vi "Z900_navX_Internal_ProcessingLoop.vi"(11 "navX Device":T1={"Interface"={"Protocol"=enum."SERIAL", "Update Rate (4Hz-60Hz)"=4, "navX Open TypeDef"=variant}, "Notify Packet"=refnum, "Loop VI Refnum"=refnum, "Ready to Close Occurrence Refnum"=refnum} {"Interface"."Update Rate (4Hz-60Hz)" min=4 max=60 step=1}) -> (0 "error out":errorcluster, 2 "Registry":u8[](array[numeric]))   [LabVIEW 2017, in "navX Library v2.lvlib"]
doc: "This navX VI handles the reading/writing for the navX. All of the good stuff is in here.\nTHIS VI SHOULD NOT BE CALLED BY THE USER!"
uses:
  navX Library v2.lvlib
  TypeDefs/Z900_navX_DeviceTypeDef.ctl
  TypeDefs/Z900_navX_ProtocolTypeDef.ctl
  TypeDefs/Z900_navX_NotifyPacketTypeDef.ctl
  TypeDefs/Z900_navX_ActionTypeDef.ctl
  <vilib>/Platform/TimedLoop/XDataNode/timing_clust.ctl
  <vilib>/Platform/TimedLoop/XDataNode/nitl_modes.ctl
  <vilib>/Platform/TimedLoop/XDataNode/wakeup.ctl
  TypeDefs/navX Open TypeDefs/Z900_navX_OpenTypeDef_Serial.ctl
  NI WPI/WPI_SerialPort_USB.ctl
  TypeDefs/Z900_navX_SerialStreamTypeDef.ctl
  TypeDefs/Z900_navX_ZeroVectorTypeDef.ctl
  TypeDefs/Z900_navX_DeviceRegisters.ctl
  TypeDefs/Flags/Z900_navX_Flags_CapabilityTypeDef.ctl
  <vilib>/Rock Robotics/SystemInterfaces/Utilities/FPGA_UtilitiesRead LocalTime.vi
  <vilib>/Platform/TimedLoop/XDataNode/XDataNode.xnode
  <vilib>/Platform/TimedLoop/XDataNode/XDNodeRunTimeDep.lvlib
  NI WPI/NI WPI Serial USB.lvlib
panel:
  out "Connected":bool
  in  "Halt":bool
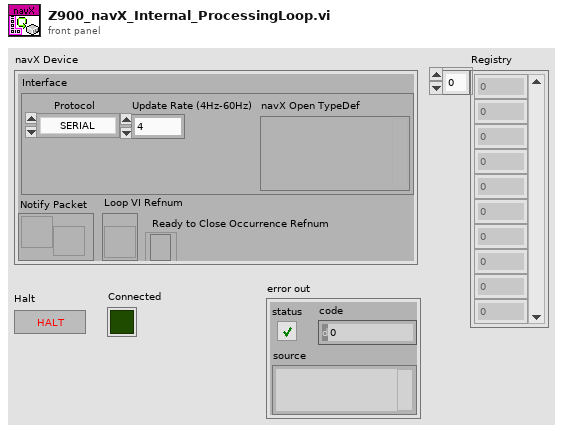
[diagram p1: front panel]
types:
  T1 = typedef "navX Library v2.lvlib/Z900_navX_DeviceTypeDef.ctl" = cluster{"Interface":cluster{"Protocol":T2, "Update Rate (4Hz-60Hz)":u8, "navX Open TypeDef":variant}, "Notify Packet":refnum<notifier>, "Loop VI Refnum":refnum<vi>, "Ready to Close Occurrence Refnum":refnum<k4>}
  T2 = typedef "navX Library v2.lvlib/Z900_navX_ProtocolTypeDef.ctl" = enum16{"SERIAL", "I2C", "SPI"}
  T3 = typedef "navX Library v2.lvlib/Z900_navX_InterfaceTypeDef.ctl" = cluster{"SerialPortRef":T4, "I2CDevRef":T5, "SPIDevRef":T7}
  T4 = typedef "WPI_SerialPortRef.ctl" = cluster{"DevStatus":errorcluster, "Serial Port Name":refnum<visa-resource-name>}
  T5 = typedef "WPI_I2CDevRef.ctl" = cluster{"DevStatus":errorcluster, "Device Address":u8, "Handle":i32, "I2C Bus":T6}
  T6 = typedef "i2c_bus.ctl" = enum16{"I2C On-Board", "I2C MXP", "Invalid"}
  T7 = typedef "WPI_SPIDevRef.ctl" = cluster{"DevStatus":errorcluster, "Handle":i32, "SPI Bus":T8}
  T8 = typedef "spi_bus.ctl" = enum16{"SPI On-Board, CS0", "SPI On-Board, CS1", "SPI On-Board, CS2", "SPI On-Board, CS3", "SPI MXP", "Invalid"}
  T9 = cluster{"Last Valid FPGA Time":dbl, "Error Count":i32, "Initialized":bool}
  T10 = typedef "XDNodeRunTimeDep.lvlib/timing_clust.ctl" = cluster{"Expected End [f-1]":u64, "Actual End [f-1]":u64, "Finished Late? [f-1]":bool, "Expected End [i-1]":u64, "Actual End [i-1]":u64, "Finished Late? [i-1]":bool, "Expected Start [i]":u64, "Actual Start [i]":u64, "Expected Start [f]":u64, "Actual Start [f]":u64, "Source Name":string, "Structure Name":string, "Period":i64, "Deadline":i64, "Offset":i64, "Start":i64, "Priority":i32, "Timeout":i32, "Mode":T11, "Wakeup Reason":T12, "Error":errorcluster, "Source Type":string, "Secondary Source Type":string, "Global End Time":u64, "Global Start Time":u64, "Frame Duration":u64, "Iteration Duration":u64, "Assigned CPU":i32, "I/O Scan Engine Mode":u32}
  T11 = typedef "XDNodeRunTimeDep.lvlib/nitl_modes.ctl" = enum32{"No Change", "Process missed periods, maintain original phase", "Discard missed periods, maintain original phase", "Process missed periods, ignore original phase", "Discard missed periods, ignore original phase"}
  T12 = typedef "XDNodeRunTimeDep.lvlib/wakeup.ctl" = enum32{"Normal", "Aborted", "Asynchronous wakeup", "Timing source error", "Timed loop error", "Timeout"}
  T13 = typedef "navX Library v2.lvlib/Z900_navX_OpenTypeDef_Serial.ctl" = cluster{"Serial Port":T14, "Stream Type":T15}
  T14 = typedef "NI WPI Serial USB.lvlib/WPI_SerialPort_USB.ctl" = enum16{"Onboard RS-232", "MXP TTL", "USB"}
  T15 = typedef "navX Library v2.lvlib/Z900_navX_SerialStreamTypeDef.ctl" = enum16{"YRPH", "Quaterinons", "Gyro/Raw", "AHRS", "AHRSAndPositioning"}
  T16 = typedef "navX Library v2.lvlib/Z900_navX_ZeroVectorTypeDef.ctl" = cluster{"X":bool, "Y":bool, "Z":bool}
  T17 = typedef "navX Library v2.lvlib/Z900_navX_NotifyPacketTypeDef.ctl" = cluster{"navX Action":T18, "Data":variant}
  T18 = typedef "navX Library v2.lvlib/Z900_navX_ActionTypeDef.ctl" = enum16{"None", "Halt", "Update Serial Protocol", "Zero-Yaw", "Zero-Displacement", "Zero-Velocity"}
  T19 = typedef "navX Library v2.lvlib/Z900_navX_DeviceRegisters.ctl" = u8
  T20 = typedef "navX Library v2.lvlib/Z900_navX_Flags_CapabilityTypeDef.ctl" = u16
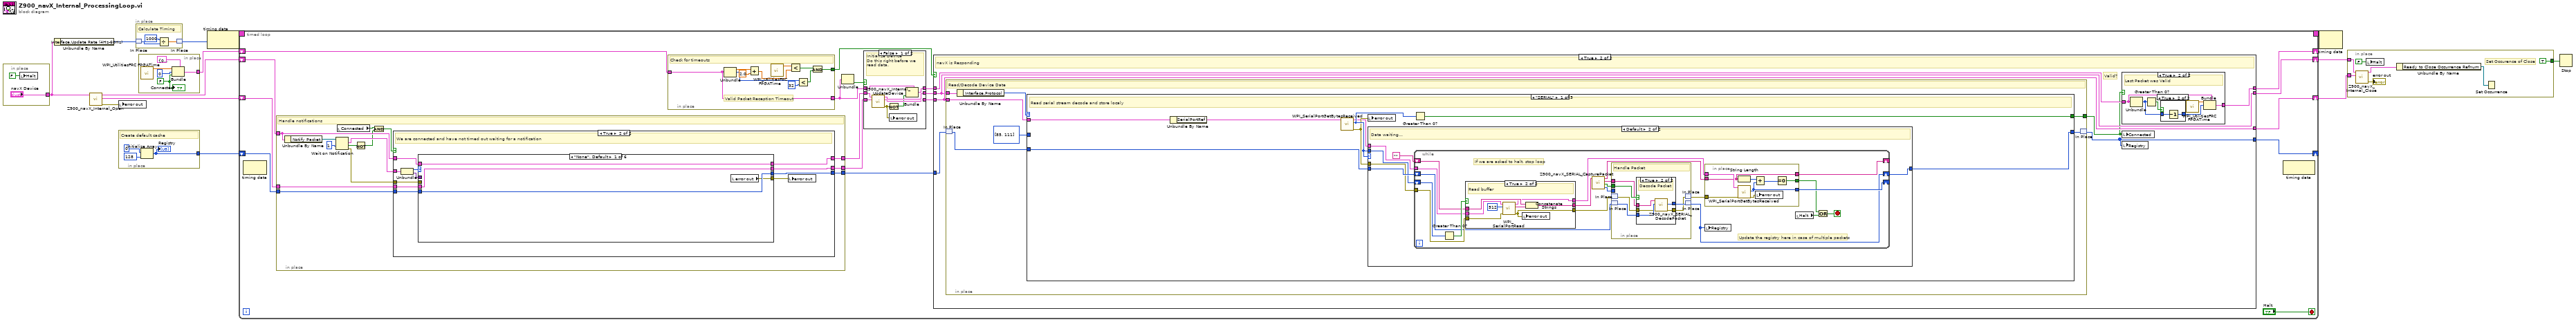
[diagram p0: block diagram]
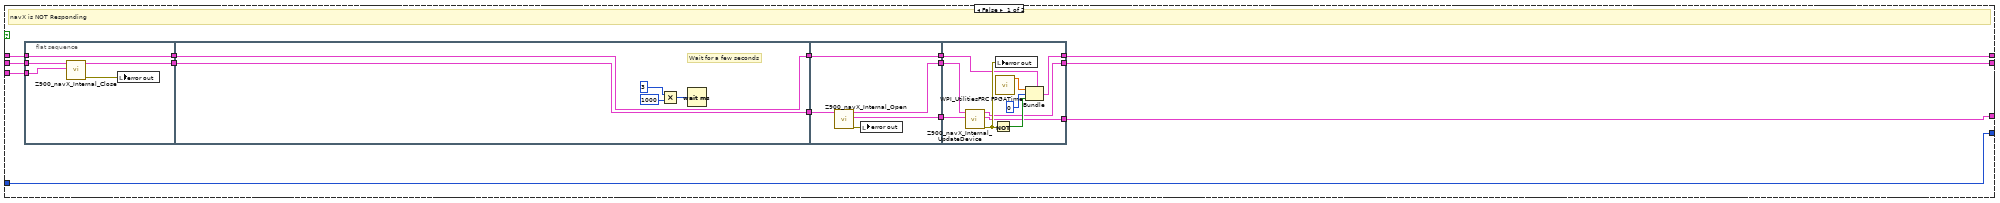
[diagram p3: hidden frame]
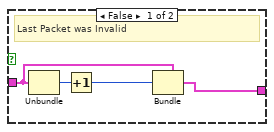
[diagram p4: hidden frame]
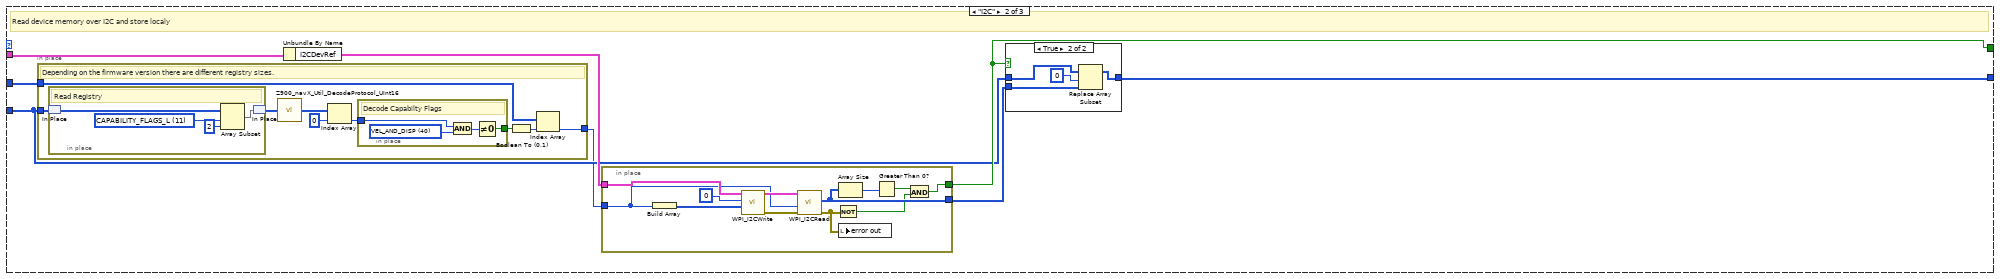
[diagram p9: hidden frame]
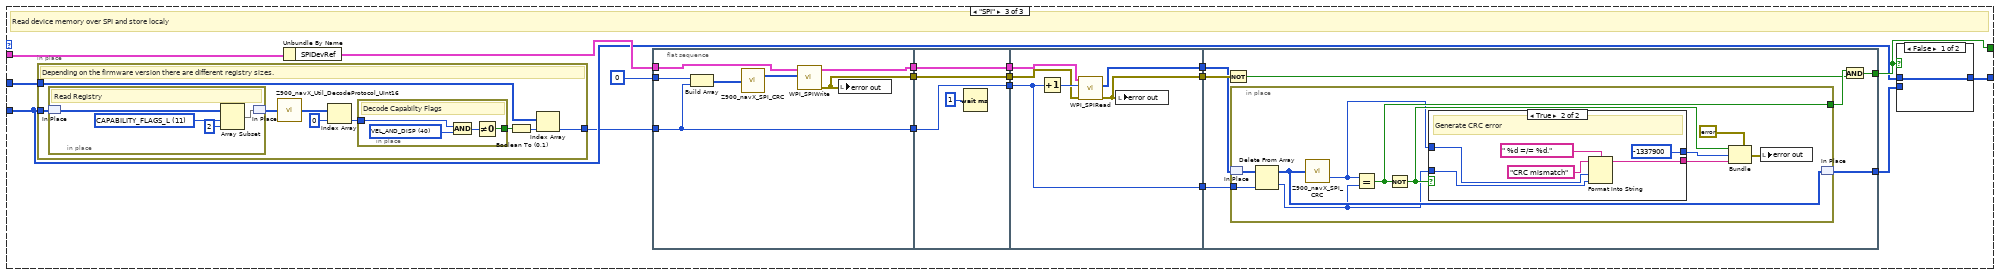
[diagram p11: hidden frame]
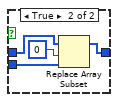
[diagram p12: hidden frame]
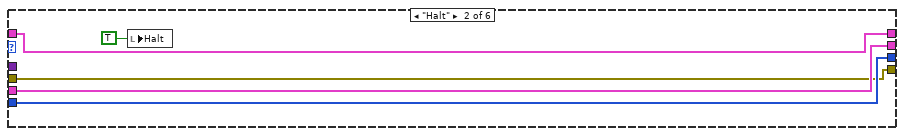
[diagram p15: hidden frame]
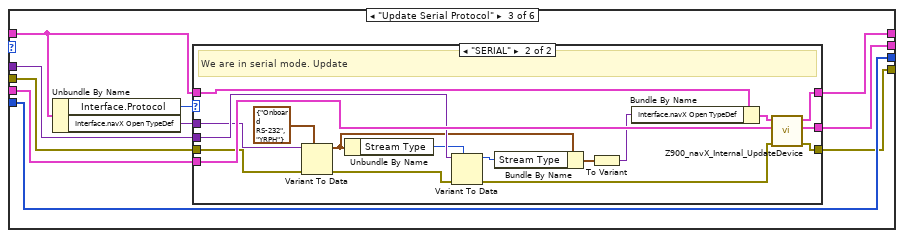
[diagram p16: hidden frame]
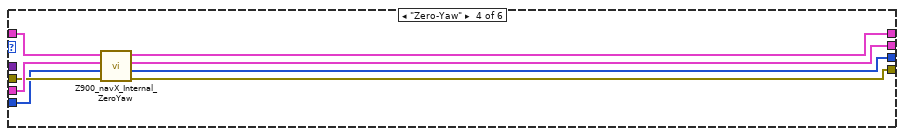
[diagram p18: hidden frame]
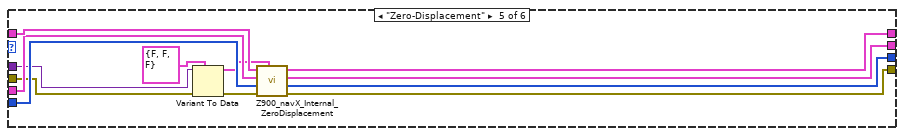
[diagram p19: hidden frame]
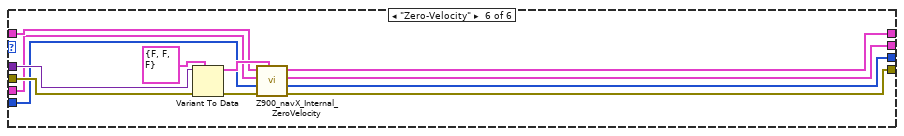
[diagram p20: hidden frame]
diagram:
  n1 = in-place {
    in-place-border: ["navX Device"] -> w6
    n2 = local write "Halt"(FALSE ("Halt")) -> ()
  }
  n3 = Unbundle By Name(w6) -> ("Interface.Update Rate (4Hz-60Hz)"=w10:u8)
  n4 = call "Z900_navX_Internal_Open.vi"("navX Device"=w6) -> ("error out"=w2:errorcluster, "Interface TypeDefs"=w5:T3, "navX Device"=w3:T1)  [unwired: 8 in]
  n5 = local write "error out"(w2) -> ()
  n6 = in-place {
    in-place-border: [w16] -> w9
    # "Create default cache"
    n7 = Initialize Array(u8 0 ("Received Data"), 128 ("hex")) -> (w16:u8[])
    "Registry" <- w16
  }
  n8 = in-place {
    # "Calculate Timing"
    n9 = in-place-match #1(w10) -> (w20:u8)
    n10 = Divide(x=1000, y=w20) -> (x/y=w19:dbl)
    n11 = in-place-match #1(w19) -> (w11:u8)
  }
  n12 = in-place {
    in-place-border: [w24] -> w4
    w22 = FALSE ("Initialized")
    n13 = call <vilib>:"WPI_UtilitiesFRC FPGATime.vi"() -> ("FPGA Time"=w25:dbl)  [unwired: 10 in, 1 out]
    n14 = Bundle(cluster=T9 {"Last Valid FPGA Time"=0.0, "Error Count"=0, "Initialized"=FALSE}, "Last Valid FPGA Time"=w25, "Error Count"=0, "Initialized"=w22) -> (w24:T9)
    "Connected" <- w22
  }
  n15 = node-c288(w11) -> (w13:T10)
  n16 = timed-loop {
    timing: w13 -> [_]
    timing-out: [_] -> w12
    shift-right: [w44] -> _
    shift-left: w9 -> [w40]
    shift-right: [w41] -> w8
    shift-left: w3 -> [w30]
    shift-right: [w42] -> w7
    shift-left: w5 -> [w29]
    shift-right: [w43] -> _
    shift-left: w4 -> [w27]
    stop <- "Halt" stop-if-true
    n17 = node-c288() -> ()  [unwired: 1 in, 1 out]
    n18 = in-place {
      in-place-border: w30 -> [w332]
      in-place-border: w29 -> [w331]
      in-place-border: [w330] -> w33
      in-place-border: [w329] -> w34
      in-place-border: w40 -> [w327]
      in-place-border: [w326] -> w39
      # "Handle notifications"
      n19 = Unbundle By Name(w332) -> ("Notify Packet"=w334:refnum<notifier>)
      n20 = Wait on Notification(notifier=w334, timeout in ms (-1)=1) -> (notification=w335:T17, timed out?=w325:bool, error out=w328:errorcluster)  [unwired: 2 in, 1 out]
      n21 = local read "Connected"() -> (w323:bool)
      n22 = Not(x=w325) -> (.not. x?=w324:bool)
      n23 = And(x=w323, y=w324) -> (x .and. y?=w322:bool)
      n24 = case shown="True" w322 {
        tunnel: w335 -> [_ w349]
        tunnel: w332 -> [w338 w347]
        tunnel: w331 -> [w337 w346]
        tunnel: [w337 w345] -> w330
        tunnel: [w338 w344] -> w329
        tunnel: w328 -> [_ w342]
        tunnel: w327 -> [w336 w341]
        tunnel: [w336 w340] -> w326
        frame False {
          # "We are either not connected or have timed out waiting for a notification"
        }
        frame True {
          # "We are connected and have not timed out waiting for a notification"
          n25 = Unbundle(w349) -> ("navX Action"=w348:T18, "Data"=w343:variant)
          n26 = case shown="\"None\", Default" w348 {
            tunnel: w347 -> [w353 w358 w362 w396 w408 w415]
            tunnel: w346 -> [w352 w357 w368 w394 w406 w414]
            tunnel: [w352 w357 w367 w393 w404 w411] -> w345
            tunnel: [w353 w358 w366 w395 w405 w412] -> w344
            tunnel: w343 -> [_ _ w365 _ w401 w418]
            tunnel: w342 -> [_ w355 w363 w392 w398 w419]
            tunnel: w341 -> [w351 w356 w361 w391 w407 w413]
            tunnel: [w351 w356 w361 w390 w403 w410] -> w340
            tunnel: [w350 w355 w360 w389 w402 w409] -> w339
            frame "None", Default {
              n27 = local read "error out"() -> (w350:errorcluster)
            }
            frame "Halt" {
              n28 = local write "Halt"(TRUE) -> ()
            }
            frame "Update Serial Protocol" {
              n29 = Unbundle By Name(w362) -> ("Interface.Protocol"=w359:T2, "Interface.navX Open TypeDef"=w364:variant)
              n30 = case shown="\"SERIAL\"" w359 {
                tunnel: w368 -> [w370 w388]
                tunnel: [w370 w387] -> w367
                tunnel: [w371 w386] -> w366
                tunnel: w365 -> [_ w385]
                tunnel: w364 -> [_ w382]
                tunnel: w363 -> [w369 w379]
                tunnel: w362 -> [w371 w378]
                tunnel: [w369 w372] -> w360
                frame Default {
                  # "We don't care if we are not in serial mode."
                }
                frame "SERIAL" {
                  # "We are in serial mode. Update"
                  n31 = Variant To Data(error in=w379, type=T13 {"Serial Port"=enum."Onboard RS-232", "Stream Type"=enum."YRPH"} ("navX Serial Open"), Variant=w382) -> (data=w375:T13, error out=w380:errorcluster)
                  n32 = Unbundle By Name(w375) -> ("Stream Type"=w374:T15)
                  n33 = Variant To Data(error in=w380, type=w374, Variant=w385) -> (data=w373:T15, error out=w384:errorcluster)
                  n34 = Bundle By Name(cluster=w375, "Stream Type"=w373) -> (w383:T13)
                  n35 = To Variant(anything=w383) -> (Variant=w377:variant)
                  n36 = Bundle By Name(cluster=w378, "Interface.navX Open TypeDef"=w377) -> (w376:T1)
                  n37 = call "Z900_navX_Internal_UpdateDevice.vi"("error in (no error)"=w384, "Interface TypeDefs"=w388, "navX Device"=w376) -> ("error out"=w372:errorcluster, "Interface TypeDefs"=w387:T3, "navX Device"=w386:T1)  [unwired: 6 in]
                }
              }
            }
            frame "Zero-Yaw" {
              n38 = call "Z900_navX_Internal_ZeroYaw.vi"("error in (no error)"=w392, "Registry"=w391, "Interface TypeDefs"=w394, "navX Device"=w396) -> ("error out"=w389:errorcluster, "Registry"=w390:u8[], "Interface TypeDefs"=w393:T3, "navX Device"=w395:T1)  [unwired: 4 in]
            }
            frame "Zero-Displacement" {
              n39 = Variant To Data(error in=w398, type=T16 {"X"=FALSE, "Y"=FALSE, "Z"=FALSE} ("Zero Vector"), Variant=w401) -> (data=w399:T16, error out=w397:errorcluster)
              n40 = call "Z900_navX_Internal_ZeroDisplacement.vi"("Zero Vector"=w399, "error in (no error)"=w397, "Registry"=w407, "Interface TypeDefs"=w406, "navX Device"=w408) -> ("error out"=w402:errorcluster, "Registry"=w403:u8[], "Interface TypeDefs"=w404:T3, "navX Device"=w405:T1)  [unwired: 3 in]
            }
            frame "Zero-Velocity" {
              n41 = Variant To Data(error in=w419, type=T16 {"X"=FALSE, "Y"=FALSE, "Z"=FALSE} ("Zero Vector"), Variant=w418) -> (data=w417:T16, error out=w416:errorcluster)
              n42 = call "Z900_navX_Internal_ZeroVelocity.vi"("Zero Vector"=w417, "error in (no error)"=w416, "Registry"=w413, "Interface TypeDefs"=w414, "navX Device"=w415) -> ("error out"=w409:errorcluster, "Registry"=w410:u8[], "Interface TypeDefs"=w411:T3, "navX Device"=w412:T1)  [unwired: 3 in]
            }
          }
          n43 = local write "error out"(w339) -> ()
        }
      }
    }
    n44 = in-place {
      in-place-border: w27 -> [w56]
      in-place-border: [w57] -> w38
      in-place-border: [w56] -> w28
      # "Valid Packet Reception Timeout"
      # "Check for timeouts"
      n45 = Unbundle(w56) -> ("Last Valid FPGA Time"=w65:dbl, "Error Count"=w61:i32)  [unwired: 1 out]
      n46 = Add(x=w65, y=2.0) -> (x+y=w63:dbl)
      n47 = call <vilib>:"WPI_UtilitiesFRC FPGATime.vi"() -> ("FPGA Time"=w62:dbl)  [unwired: 10 in, 1 out]
      n48 = Less?(x=w62, y=w63) -> (x < y?=w59:bool)
      n49 = Less?(x=w61, y=32) -> (x < y?=w58:bool)
      n50 = And(x=w59, y=w58) -> (x .and. y?=w57:bool)
    }
    n51 = Unbundle(w28) -> ("Initialized"=w36:bool)  [unwired: 2 out]
    n52 = case shown="False" w36 {
      tunnel: w28 -> [w52 w55]
      tunnel: [w51 w55] -> w35
      tunnel: w34 -> [w50 w54]
      tunnel: w33 -> [w49 w53]
      tunnel: [w48 w54] -> w31
      tunnel: [w47 w53] -> w32
      frame False {
        # "Initialize Device\nDo this right before we\nread data."
        n53 = call "Z900_navX_Internal_UpdateDevice.vi"("Interface TypeDefs"=w49, "navX Device"=w50) -> ("error out"=w46:errorcluster, "Interface TypeDefs"=w47:T3, "navX Device"=w48:T1)  [unwired: 7 in]
        n54 = Not(x=w46) -> (.not. x?=w45:bool)
        n55 = local write "error out"(w46) -> ()
        n56 = Bundle(cluster=w52, "Initialized"=w45) -> (w51:T9)  [unwired: 2 in]
      }
      frame True {
      }
    }
    n57 = case shown="True" w38 {
      tunnel: w39 -> [w77 w111]
      tunnel: w32 -> [w78 w110]
      tunnel: [w77 w107] -> w44
      tunnel: w35 -> [w66 w109]
      tunnel: [w70 w108] -> w43
      tunnel: w31 -> [w79 w106]
      tunnel: [w71 w106] -> w41
      tunnel: [w74 w110] -> w42
      frame False {
        # "navX is NOT Responding"
        n58 = flat-sequence {
          tunnel: w79 -> [w82]
          tunnel: w78 -> [w84]
          tunnel: [w83] -> w76
          tunnel: [w80] -> w67
          tunnel: w66 -> [w80]
          tunnel: w76 -> [w89]
          tunnel: [w89] -> w75
          tunnel: [w85] -> w68
          tunnel: w67 -> [w85]
          tunnel: w75 -> [w93]
          tunnel: [w94] -> w73
          tunnel: [w92] -> w72
          tunnel: [w90] -> w69
          tunnel: w68 -> [w90]
          tunnel: [w102] -> w70
          tunnel: [w98] -> w74
          tunnel: [w99] -> w71
          tunnel: w69 -> [w97]
          tunnel: w72 -> [w100]
          tunnel: w73 -> [w101]
          frame #0 {
            n59 = call "Z900_navX_Internal_Close.vi"("Interface TypeDefs"=w84, "navX Device"=w82) -> ("error out"=w81:errorcluster, "navX Device"=w83:T1)  [unwired: 8 in]
            n60 = local write "error out"(w81) -> ()
          }
          frame #1 {
            # "Wait for a few seconds"
            n61 = Multiply(x=u32 3 ("milliseconds to wait"), y=u32 1000) -> (x*y=w87:u32)
            n62 = Wait (ms)(milliseconds to wait=w87) -> ()  [unwired: 1 out]
          }
          frame #2 {
            n63 = call "Z900_navX_Internal_Open.vi"("navX Device"=w93) -> ("error out"=w91:errorcluster, "Interface TypeDefs"=w92:T3, "navX Device"=w94:T1)  [unwired: 8 in]
            n64 = local write "error out"(w91) -> ()
          }
          frame #3 {
            n65 = call "Z900_navX_Internal_UpdateDevice.vi"("Interface TypeDefs"=w100, "navX Device"=w101) -> ("error out"=w103:errorcluster, "Interface TypeDefs"=w98:T3, "navX Device"=w99:T1)  [unwired: 7 in]
            n66 = Not(x=w103) -> (.not. x?=w104:bool)
            n67 = local write "error out"(w103) -> ()
            n68 = call <vilib>:"WPI_UtilitiesFRC FPGATime.vi"() -> ("FPGA Time"=w96:dbl)  [unwired: 10 in, 1 out]
            n69 = Bundle(cluster=w97, "Last Valid FPGA Time"=w96, "Error Count"=0, "Initialized"=w104) -> (w102:T9)
          }
        }
      }
      frame True {
        # "Valid?"
        # "navX is Responding"
        n70 = in-place {
          in-place-border: w106 -> [w126]
          in-place-border: w110 -> [w130]
          in-place-border: [w128] -> w105
          # "Read/Decode Device Date"
          n71 = in-place-match #2(w111) -> (w129:u8[])
          n72 = Unbundle By Name(w126) -> ("Interface.Protocol"=w131:T2)
          n73 = case shown="\"SERIAL\"" w131 {
            tunnel: [w137 w204 w251] -> w127
            tunnel: w129 -> [w138 w201 w243]
            tunnel: w130 -> [w139 w206 w258]
            tunnel: [w135 w203 w248] -> w128
            tunnel: i32[] [85, 111] -> [_ w200 w242]
            frame "SERIAL" {
              # "Read serial stream decode and store localy"
              n74 = Unbundle By Name(w139) -> ("SerialPortRef"=w136:T4)
              n75 = call <vilib>:"WPI_SerialPortGetBytesReceived.vi"("SerialPortRef"=w136) -> ("error out"=w133:errorcluster, "Bytes at Port"=w134:u32, "SerialPortRef"=w132:T4)  [unwired: 8 in]
              n76 = local write "error out"(w133) -> ()
              n77 = case shown="Default" w134 {
                tunnel: [w140 w146] -> w137
                tunnel: w138 -> [w140 w145]
                tunnel: w134 -> [_ w144]
                tunnel: w132 -> [_ w142]
                tunnel: w133 -> [_ w141]
                frame 0 {
                }
                frame Default {
                  # "Data waiting..."
                  n78 = while {
                    shift-right: [w148] -> w146
                    shift-left: w145 -> [w155]
                    shift-right: [w159] -> _
                    shift-left: w144 -> [w166]
                    shift-right: [w158] -> _
                    shift-left: "" -> [w164]
                    tunnel: w142 -> [w163]
                    tunnel: w141 -> [w162]
                    stop <- w151 stop-if-true
                    # "Update the registry here in case of multiple packets"
                    # "If we are asked to halt, stop loop"
                    n79 = Greater Than 0?(x=w166) -> (x > 0?=w165:bool)
                    n80 = case shown="True" w165 {
                      tunnel: w164 -> [w190 w198]
                      tunnel: w163 -> [w189 w197]
                      tunnel: w162 -> [w188 w194]
                      tunnel: [w190 w193] -> w161
                      tunnel: [w189 w192] -> w147
                      tunnel: [w188 w191] -> w154
                      frame False {
                        # "Pass existing buffer"
                      }
                      frame True {
                        # "Read buffer"
                        n81 = call <vilib>:"WPI_SerialPortRead.vi"("error in (no error)"=w194, "Num Bytes to Read"=u32 512, "SerialPortRef"=w197) -> ("error out"=w191:errorcluster, "Buffer"=w196:string, "SerialPortRef"=w192:T4)  [unwired: 6 in]
                        n82 = local write "error out"(w191) -> ()
                        n83 = Concatenate Strings(w198, w196) -> (w193:string)
                      }
                    }
                    n84 = call "Z900_navX_SERIAL_CapturePacket.vi"("Buffer"=w161) -> ("Packet Size"=w156:i32, "Packet Located"=w149:bool, "Packet"=w157:string, "Buffer"=w160:string)  [unwired: 7 in]
                    n85 = in-place {
                      in-place-border: w157 -> [w171]
                      in-place-border: w149 -> [w172]
                      in-place-border: w156 -> [_]
                      # "Handle Packet"
                      n86 = in-place-match #3(w154) -> (w168:errorcluster)
                      n87 = in-place-match #4(w155) -> (w169:u8[])
                      n88 = case shown="True" w172 {
                        tunnel: w171 -> [_ w179]
                        tunnel: [w174 w177] -> w170
                        tunnel: w169 -> [w174 w178]
                        tunnel: w168 -> [w173 w176]
                        tunnel: [w173 w175] -> w167
                        frame False {
                          # "No Packet"
                        }
                        frame True {
                          # "Decode Packet"
                          n89 = call "Z900_navX_SERIAL_DecodePacket.vi"("error in (no error)"=w176, "Data"=w178, "Packet"=w179) -> ("error out"=w175:errorcluster, "Data"=w177:u8[])  [unwired: 6 in, 1 out]
                        }
                      }
                      n90 = in-place-match #3(w167) -> (w153:errorcluster)
                      n91 = in-place-match #4(w170) -> (w148:u8[])
                    }
                    n92 = in-place {
                      in-place-border: w147 -> [w187]
                      in-place-border: w153 -> [w186]
                      in-place-border: w160 -> [w181]
                      in-place-border: [w183] -> w152
                      in-place-border: [w182] -> w159
                      in-place-border: [w181] -> w158
                      n93 = String Length(string=w181) -> (length=w184:i32)
                      n94 = call <vilib>:"WPI_SerialPortGetBytesReceived.vi"("error in (no error)"=w186, "SerialPortRef"=w187) -> ("error out"=w180:errorcluster, "Bytes at Port"=w182:u32)  [unwired: 7 in, 1 out]
                      n95 = Add(x=w184, y=w182) -> (x+y=w185:u32)
                      n96 = local write "error out"(w180) -> ()
                      n97 = Equal To 0?(x=w185) -> (x = 0?=w183:bool)
                    }
                    n98 = local write "Registry"(w148) -> ()
                    n99 = local read "Halt"() -> (w150:bool)
                    n100 = Or(x=w152, y=w150) -> (x .or. y?=w151:bool)
                  }
                }
              }
              n101 = Greater Than 0?(x=w134) -> (x > 0?=w135:bool)
            }
            frame "I2C" {
              # "Read device memory over I2C and store localy"
              n102 = in-place {
                in-place-border: w201 -> [w215]
                in-place-border: w200 -> [w208]
                in-place-border: [w207] -> w199
                # "Depending on the firmware version there are different registry sizes."
                n103 = in-place {
                  w223 = T19 11 items=["WHOAMI"=0, "HW_REV"=1, "FW_VER_MAJOR"=2, "FW_VER_MINOR"=3, "UPDATE_RATE_HZ"=4, "ACCEL_FSR_G"=5, "GYRO_FSR_DPS"=6, "OP_STATUS"=8, "CAL_STATUS"=9, "SELFTEST_STATUS"=10, "CAPABILITY_FLAGS_L"=11, "CAPABILITY_FLAGS_H"=12, "SENSOR_STATUS"=16, "TIMESTAMP"=18, "YAW"=22, "ROLL"=24, "PITCH"=26, "HEADING"=28, "FUSED_HEADING"=30, "ALTITUDE_I"=32, "ALTITUDE_D"=34, "LINERA_ACC_X"=36, "LINERA_ACC_Y"=38, "LINERA_ACC_Z"=40, "QUAT_W"=42, "QUAT_X"=44, "QUAT_Y"=46, "QUAT_Z"=48, "MPU_TEMP_C"=50, "GYRO_X"=52, "GYRO_Y"=54, "GYRO_Z"=56, "ACC_X"=58, "ACC_Y"=60, "ACC_Z"=62, "MAG_X"=64, "MAG_Y"=66, "MAG_Z"=68, "PRESSURE_I"=70, "PRESSURE_D"=72, "PRESSURE_TEMP"=74, "YAW_OFFSET"=76, "QUAT_OFFSET_W"=78, "QUAT_OFFSET_X"=80, "QUAT_OFFSET_Y"=82, "QUAT_OFFSET_Z"=84, "INTEGRATION_CONTROL"=86, "VELOCITY_X"=88, "VELOCITY_Y"=92, "VELOCITY_Z"=96, "DISPLACMENT_X"=100, "DISPLACMENT_Y"=104, "DISPLACEMENT_Z"=108] ("Device Register")
                  # "Read Registry"
                  n104 = in-place-match #5(w215) -> (w221:u8[])
                  n105 = Array Subset(array=w221, index=w223, length=2) -> (w222:u8[])
                  n106 = in-place-match #5(w222) -> (w212:u8[])
                }
                n107 = call "Z900_navX_Util_DecodeProtocol_UInt16.vi"("Little Endian"=w212) -> ("UInt16"=w213:u16[])
                n108 = Index Array(array=w213, index=0) -> (element=w211:u16)
                n109 = in-place {
                  in-place-border: w211 -> [w217]
                  in-place-border: [w216] -> w210
                  w219 = T20 40 items=["OMNIMOUNT"=4, "OMNIMOUNT_CONFIG_MASK"=38, "VEL_AND_DISP"=40, "YAW_RESET"=80] ("Capability Flag")
                  # "Decode Capabilty Flags"
                  n110 = And(x=w217, y=w219) -> (x .and. y?=w218:T20)
                  n111 = Not Equal To 0?(x=w218) -> (x != 0?=w216:bool)
                }
                n112 = Boolean To (0,1)(Boolean=w210) -> (0, 1=w209:i16)
                n113 = Index Array(array=w208, index=w209) -> (element=w207:i32)
              }
              n114 = Unbundle By Name(w206) -> ("I2CDevRef"=w202:T5)
              n115 = in-place {
                in-place-border: [w229] -> w205
                in-place-border: [w228] -> w203
                in-place-border: w202 -> [w226]
                in-place-border: w199 -> [w224]
                n116 = Build Array(w224) -> (w235:i32[])
                n117 = call <vilib>:"WPI_I2CWrite.vi"("I2CDataToSend"=w235, "I2CRegister"=u8 0 ("hex"), "I2CDevRef"=w226) -> ("error out"=w234:errorcluster, "I2CDevRef"=w233:T5)  [unwired: 7 in]
                n118 = call <vilib>:"WPI_I2CRead.vi"("error in (no error)"=w234, "I2CBytesToRead"=w224, "I2CDevRef"=w233) -> ("error out"=w225:errorcluster, "Data Out"=w229:u8[])  [unwired: 6 in, 1 out]
                n119 = Not(x=w225) -> (.not. x?=w227:bool)
                n120 = Array Size(array=w229) -> (size(s)=w231:i32)
                n121 = local write "error out"(w225) -> ()
                n122 = Greater Than 0?(x=w231) -> (x > 0?=w230:bool)
                n123 = And(x=w230, y=w227) -> (x .and. y?=w228:bool)
              }
              n124 = case shown="True" w203 {
                tunnel: w201 -> [w236 w240]
                tunnel: [w236 w239] -> w204
                tunnel: w205 -> [_ w238]
                frame False {
                }
                frame True {
                  n125 = Replace Array Subset(array=w240, new element=w238, index=u8 0 ("hex")) -> (w239:u8[])
                }
              }
            }
            frame "SPI" {
              # "Read device memory over SPI and store localy"
              n126 = in-place {
                in-place-border: w243 -> [w267]
                in-place-border: w242 -> [w260]
                in-place-border: [w259] -> w241
                # "Depending on the firmware version there are different registry sizes."
                n127 = in-place {
                  w275 = T19 11 items=["WHOAMI"=0, "HW_REV"=1, "FW_VER_MAJOR"=2, "FW_VER_MINOR"=3, "UPDATE_RATE_HZ"=4, "ACCEL_FSR_G"=5, "GYRO_FSR_DPS"=6, "OP_STATUS"=8, "CAL_STATUS"=9, "SELFTEST_STATUS"=10, "CAPABILITY_FLAGS_L"=11, "CAPABILITY_FLAGS_H"=12, "SENSOR_STATUS"=16, "TIMESTAMP"=18, "YAW"=22, "ROLL"=24, "PITCH"=26, "HEADING"=28, "FUSED_HEADING"=30, "ALTITUDE_I"=32, "ALTITUDE_D"=34, "LINERA_ACC_X"=36, "LINERA_ACC_Y"=38, "LINERA_ACC_Z"=40, "QUAT_W"=42, "QUAT_X"=44, "QUAT_Y"=46, "QUAT_Z"=48, "MPU_TEMP_C"=50, "GYRO_X"=52, "GYRO_Y"=54, "GYRO_Z"=56, "ACC_X"=58, "ACC_Y"=60, "ACC_Z"=62, "MAG_X"=64, "MAG_Y"=66, "MAG_Z"=68, "PRESSURE_I"=70, "PRESSURE_D"=72, "PRESSURE_TEMP"=74, "YAW_OFFSET"=76, "QUAT_OFFSET_W"=78, "QUAT_OFFSET_X"=80, "QUAT_OFFSET_Y"=82, "QUAT_OFFSET_Z"=84, "INTEGRATION_CONTROL"=86, "VELOCITY_X"=88, "VELOCITY_Y"=92, "VELOCITY_Z"=96, "DISPLACMENT_X"=100, "DISPLACMENT_Y"=104, "DISPLACEMENT_Z"=108] ("Device Register")
                  # "Read Registry"
                  n128 = in-place-match #6(w267) -> (w273:u8[])
                  n129 = Array Subset(array=w273, index=w275, length=2) -> (w274:u8[])
                  n130 = in-place-match #6(w274) -> (w264:u8[])
                }
                n131 = call "Z900_navX_Util_DecodeProtocol_UInt16.vi"("Little Endian"=w264) -> ("UInt16"=w265:u16[])
                n132 = Index Array(array=w265, index=0) -> (element=w263:u16)
                n133 = in-place {
                  in-place-border: w263 -> [w269]
                  in-place-border: [w268] -> w262
                  w271 = T20 40 items=["OMNIMOUNT"=4, "OMNIMOUNT_CONFIG_MASK"=38, "VEL_AND_DISP"=40, "YAW_RESET"=80] ("Capability Flag")
                  # "Decode Capabilty Flags"
                  n134 = And(x=w269, y=w271) -> (x .and. y?=w270:T20)
                  n135 = Not Equal To 0?(x=w270) -> (x != 0?=w268:bool)
                }
                n136 = Boolean To (0,1)(Boolean=w262) -> (0, 1=w261:i16)
                n137 = Index Array(array=w260, index=w261) -> (element=w259:i32)
              }
              n138 = Unbundle By Name(w258) -> ("SPIDevRef"=w244:T7)
              n139 = flat-sequence {
                tunnel: u8 0 ("hex") -> [w287]
                tunnel: w241 -> [w282]
                tunnel: w244 -> [w284]
                tunnel: [w283] -> w257
                tunnel: [w282] -> w254
                tunnel: [w281] -> w247
                tunnel: w257 -> [w290]
                tunnel: [w290] -> w256
                tunnel: [w289] -> w255
                tunnel: w254 -> [w289]
                tunnel: w247 -> [w288]
                tunnel: [w288] -> w246
                tunnel: w256 -> [w297]
                tunnel: w255 -> [w294]
                tunnel: [w295] -> w253
                tunnel: [w294] -> w252
                tunnel: w246 -> [w293]
                tunnel: [w292] -> w245
                tunnel: w253 -> [w300]
                tunnel: w252 -> [w304]
                tunnel: [w301] -> w248
                tunnel: [w299] -> w250
                tunnel: w245 -> [w303]
                frame #0 {
                  n140 = Build Array(w287, w282) -> (w286:i32[])
                  n141 = call "Z900_navX_SPI_CRC.vi"("Message"=w286) -> ("Message with CRC"=w285:u8[])  [unwired: 1 out]
                  n142 = call <vilib>:"WPI_SPIWrite.vi"("Data To Send"=w285, "SPIDevRef"=w284) -> ("error out"=w281:errorcluster, "SPIDevRef"=w283:T7)  [unwired: 7 in, 1 out]
                  n143 = local write "error out"(w281) -> ()
                }
                frame #1 {
                  n144 = Wait (ms)(milliseconds to wait=u32 1) -> ()  [unwired: 1 out]
                }
                frame #2 {
                  n145 = Increment(x=w294) -> (x+1=w296:i32)
                  n146 = call <vilib>:"WPI_SPIRead.vi"("error in (no error)"=w293, "Num to Read"=w296, "SPIDevRef"=w297) -> ("error out"=w292:errorcluster, "Received Data"=w295:u8[])  [unwired: 6 in, 1 out]
                  n147 = local write "error out"(w292) -> ()
                }
                frame #3 {
                  n148 = Not(x=w303) -> (.not. x?=w298:bool)
                  n149 = in-place {
                    in-place-border: w304 -> [w315]
                    in-place-border: [w312] -> w302
                    n150 = in-place-match #7(w300) -> (w314:u8[])
                    n151 = Delete From Array(array=w314, index=w315) -> (deleted portion=w309:u8, array with subset deleted=w313:u8[])  [unwired: 1 in]
                    n152 = call "Z900_navX_SPI_CRC.vi"("Message"=w313) -> ("CRC"=w310:u8)  [unwired: 1 out]
                    n153 = Equal?(x=w310, y=w309) -> (x = y?=w312:bool)
                    n154 = Not(x=w312) -> (.not. x?=w311:bool)
                    n155 = case shown="True" w311 {
                      tunnel: w310 -> [_ w319]
                      tunnel: w309 -> [_ w318]
                      tunnel: [_ w317] -> w308
                      tunnel: [_ -1337900 ("code")] -> w305
                      frame False {
                      }
                      frame True {
                        # "Generate CRC error"
                        n156 = Format Into String(format string=" %d =/= %d.", initial string="CRC mismatch", w319, w318) -> (resulting string=w317:string)  [unwired: 1 in, 1 out]
                      }
                    }
                    n157 = Bundle(cluster=errorcluster {"status"=FALSE, "code"=0, "source"=""} ("error constant"), "status"=w311, "code"=w305, "source"=w308) -> (w306:errorcluster)
                    n158 = local write "error out"(w306) -> ()
                    n159 = in-place-match #7(w313) -> (w299:u8[])
                  }
                  n160 = And(x=w302, y=w298) -> (x .and. y?=w301:bool)
                }
              }
              n161 = case shown="False" w248 {
                tunnel: w243 -> [w276 w280]
                tunnel: [w276 w279] -> w251
                tunnel: w250 -> [_ w278]
                frame False {
                }
                frame True {
                  n162 = Replace Array Subset(array=w280, new element=w278, index=u8 0 ("hex")) -> (w279:u8[])
                }
              }
            }
          }
          n163 = in-place-match #2(w127) -> (w107:u8[])
        }
        n164 = case shown="True" w105 {
          tunnel: [w112 w120] -> w108
          tunnel: w109 -> [w113 w119]
          frame False {
            # "Last Packet was Invalid"
            n165 = Unbundle(w113) -> ("Error Count"=w114:i32)  [unwired: 2 out]
            n166 = Increment(x=w114) -> (x+1=w115:i32)
            n167 = Bundle(cluster=w113, "Error Count"=w115) -> (w112:T9)  [unwired: 2 in]
          }
          frame True {
            # "Last Packet was Valid"
            n168 = Unbundle(w119) -> ("Error Count"=w117:i32)  [unwired: 2 out]
            n169 = Greater Than 0?(x=w117) -> (x > 0?=w118:bool)
            n170 = case shown="True" w118 {
              tunnel: [w122 w123] -> w116
              tunnel: w117 -> [w122 w124]
              frame False {
              }
              frame True {
                n171 = Decrement(x=w124) -> (x-1=w123:i32)
              }
            }
            n172 = call <vilib>:"WPI_UtilitiesFRC FPGATime.vi"() -> ("FPGA Time"=w121:dbl)  [unwired: 10 in, 1 out]
            n173 = Bundle(cluster=w119, "Last Valid FPGA Time"=w121, "Error Count"=w116) -> (w120:T9)  [unwired: 1 in]
          }
        }
        n174 = local write "Connected"(w105) -> ()
        n175 = local write "Registry"(w107) -> ()
      }
    }
    n176 = node-c288() -> ()  [unwired: 1 in, 1 out]
  }
  n177 = node-c288(w12) -> ()  [unwired: 1 out]
  n178 = in-place {
    in-place-border: w8 -> [w429]
    in-place-border: w7 -> [w428]
    in-place-border: [TRUE] -> w1
    # "Set Occurence of Close"
    n179 = call "Z900_navX_Internal_Close.vi"("Interface TypeDefs"=w428, "navX Device"=w429) -> ("error out"=→"error out":errorcluster, "navX Device"=w423:T1)  [unwired: 8 in]
    n180 = local write "Halt"(FALSE ("Halt")) -> ()
    n181 = Unbundle By Name(w423) -> ("Ready to Close Occurrence Refnum"=w425:refnum<k4>)
    n182 = Set Occurrence(w425) -> ()
  }
  n183 = Stop(stop? (T)=w1) -> ()
